vi "Disconnect from Slave.vi"(8 "error in (no error)":errorcluster, 11 "Modbus master in":refnum<class "Modbus Master.lvclass">) -> (0 "error out":errorcluster, 3 "Modbus master out":refnum<class "Modbus Master.lvclass">)   [LabVIEW 2021, in "Modbus Master.lvclass"]
doc: "Initializes a Modbus master instance. If using the <B>Create Modbus Instance</B> VI, this is not necessary. This function will initiate any required bus communication."
uses:
  Modbus Master.lvclass
  C:/my_projects/projects/Algorithms/Labview/21/Modbus_v121c/API/Modbus API.lvclass
  Modbus Master.lvclass/Modbus Master.ctl
  Modbus API.lvclass/Modbus API.ctl
  Network Protocol/Network Master/Network Master.lvclass
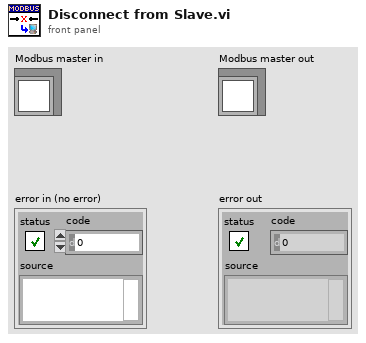
[diagram p1: front panel]
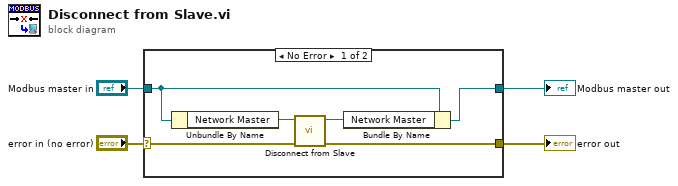
[diagram p0: block diagram]
diagram:
  n1 = case shown="No Error" "error in (no error)" {
    selector: "error in (no error)" -> [w6 w11]
    tunnel: [w9 w12] -> w2
    tunnel: "Modbus master in" -> [w10 w12]
    tunnel: [w5 w11] -> w1
    frame No Error {
      n2 = Unbundle By Name(w10) -> ("Network Master"=w8:refnum<class "Network Master.lvclass">)
      n3 = call-dynamic "Disconnect from Slave.vi"("error in (no error)"=w6, "network master in"=w8) -> ("error out"=w5:errorcluster, "network master out"=w7:refnum<class "Network Master.lvclass">)  [unwired: 8 in]
      n4 = Bundle By Name(cluster=w10, "Network Master"=w7) -> (w9:refnum<class "Modbus Master.lvclass">)
    }
    frame Error {
    }
  }
  "error out" <- w1
  "Modbus master out" <- w2
